vi "QuinticHermiteSpline_getControlVectorFromArrays.vi"(9 "finalVector":dbl[](array[numeric]), 11 "initialVector":dbl[](array[numeric])) -> (0 "error out":errorcluster, 3 "ControlVector":T1)   [LabVIEW 2019, in "Trajectory_Library.lvlib"]
doc: "Returns the control vector for each dimension as a matrix from the user-provided arrays in the constructor.\n \nParameters:\n - initialVector - The control vector for the initial point.\n - finalVector - The control vector for the final point.\n\nReturns:\n - ControlVector - The control vector matrix for a dimension.\n - Error Out - The returned error cluster"
uses:
  Trajectory_Library.lvlib
  <vilib>/Analysis/Matrix/Datatypes/RealMatrix.ctl
  <vilib>/Analysis/Matrix/NI_Matrix.lvlib
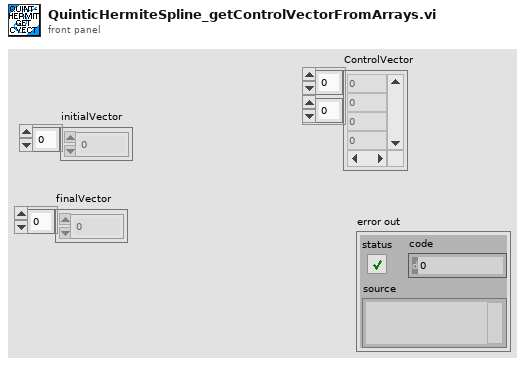
[diagram p1: front panel]
types:
  T1 = typedef "NI_Matrix.lvlib/RealMatrix.ctl" = dbl[][]
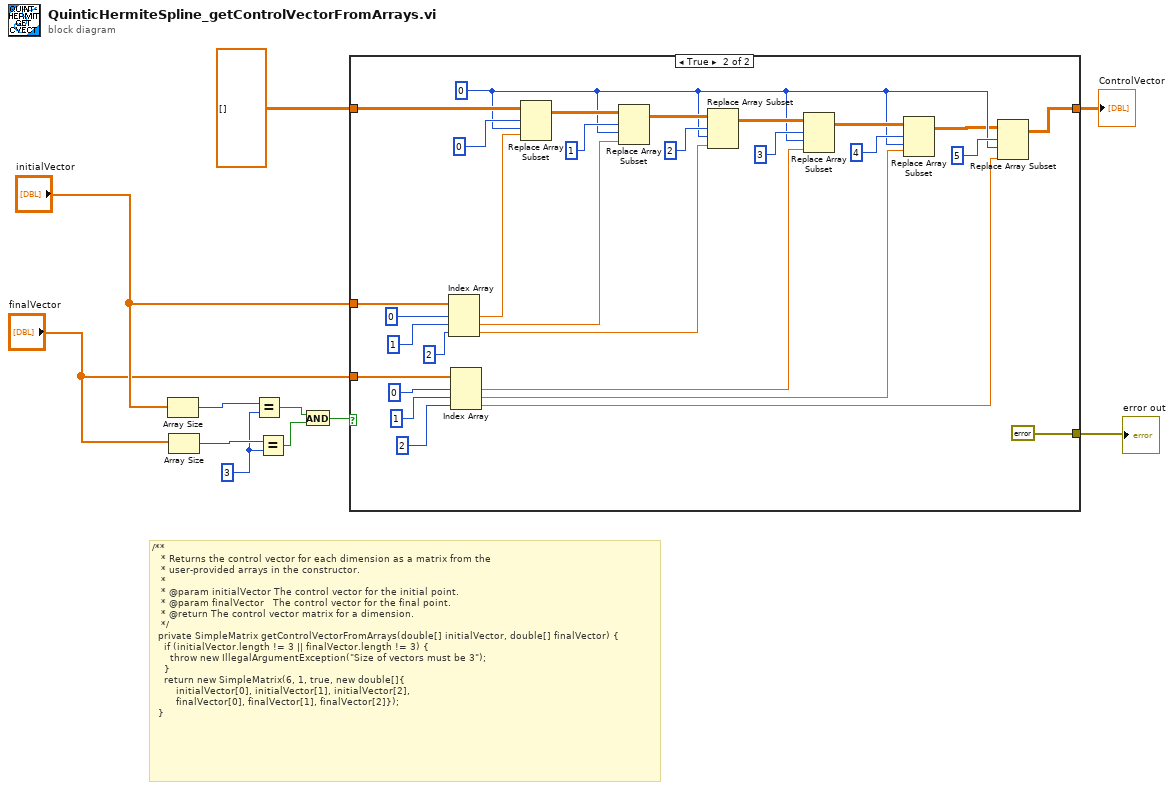
[diagram p0: block diagram]
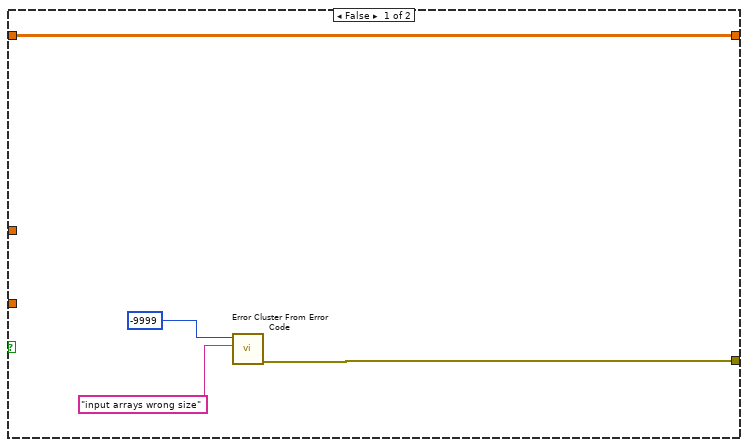
[diagram p2: hidden frame]
diagram:
  w9 = 3 ("y")
  # "/**\n   * Returns the control vector for each dimension as a matrix from the\n   * user-provided arrays in the constructor.\n   *\n   * @param initialVector The control vector for the initial point.\n   * @param finalVector   The control vector for the final point.\n   * @return The control vector matrix for a dimension.\n   */\n  private SimpleMatrix getControlVectorFromArrays(double[] initialVector, double[] finalVector) {\n    if (initialVector.length != 3 || finalVector.length != 3) {\n      throw new IllegalArgumentException(\"Size of vectors must be 3\");\n    }\n    return new SimpleMatrix(6, 1, true, new double[]{\n        initialVector[0], initialVector[1], initialVector[2],\n        finalVector[0], finalVector[1], finalVector[2]});\n  }"
  n1 = Array Size(array="initialVector") -> (size(s)=w11:i32)
  n2 = Array Size(array="finalVector") -> (size(s)=w10:i32)
  n3 = Equal?(x=w11, y=w9) -> (x = y?=w8:bool)
  n4 = Equal?(x=w10, y=w9) -> (x = y?=w7:bool)
  n5 = And(x=w8, y=w7) -> (x .and. y?=w6:bool)
  n6 = case shown="True" w6 {
    tunnel: [w15 errorcluster {"status"=FALSE, "code"=0, "source"=""} ("error out")] -> w5
    tunnel: [w12 w18] -> w4
    tunnel: T1 [] ("ControlVector") -> [w12 w43]
    tunnel: "initialVector" -> [_ w36]
    tunnel: "finalVector" -> [_ w33]
    frame False {
      n7 = call <vilib>:"Error Cluster From Error Code.vi"("error message (\"\")"="input arrays wrong size" ("error message (\"\")"), "error code (0)"=-9999) -> ("error out"=w15:errorcluster)  [unwired: 7 in]
    }
    frame True {
      w20 = 0 ("disabled index (col)")
      n8 = Index Array(array=w36, index #1=0 ("index"), index #2=1 ("index"), index #3=2 ("index")) -> (element #1=w32:dbl, element #2=w31:dbl, element #3=w25:dbl)
      n9 = Index Array(array=w33, index #1=0 ("index"), index #2=1 ("index"), index #3=2 ("index")) -> (element #1=w30:dbl, element #2=w29:dbl, element #3=w21:dbl)
      n10 = Replace Array Subset(array=w43, new element=w32, index (row)=0 ("disabled index (row)"), index (col)=w20) -> (w41:T1)
      n11 = Replace Array Subset(array=w41, new element=w31, index (row)=1 ("disabled index (row)"), index (col)=w20) -> (w24:T1)
      n12 = Replace Array Subset(array=w24, new element=w25, index (row)=2 ("disabled index (row)"), index (col)=w20) -> (w23:T1)
      n13 = Replace Array Subset(array=w23, new element=w30, index (row)=3 ("disabled index (row)"), index (col)=w20) -> (w40:T1)
      n14 = Replace Array Subset(array=w40, new element=w29, index (row)=4 ("disabled index (row)"), index (col)=w20) -> (w19:T1)
      n15 = Replace Array Subset(array=w19, new element=w21, index (row)=5 ("disabled index (row)"), index (col)=w20) -> (w18:T1)
    }
  }
  "ControlVector" <- w4
  "error out" <- w5
